vi "Autonomous Motor Input.vi"(0 "RotationTarget":dbl, 1 "Y_axis":dbl, 2 "X_axis":dbl, 5 "Squeeze":dbl, 7 "Cluster in":T1, 9 "Arms":dbl, 12 "ArmLift":dbl, 13 "Hands":dbl, 14 "Lift":dbl) -> (4 "Cluster out":T1)   [LabVIEW 2017]
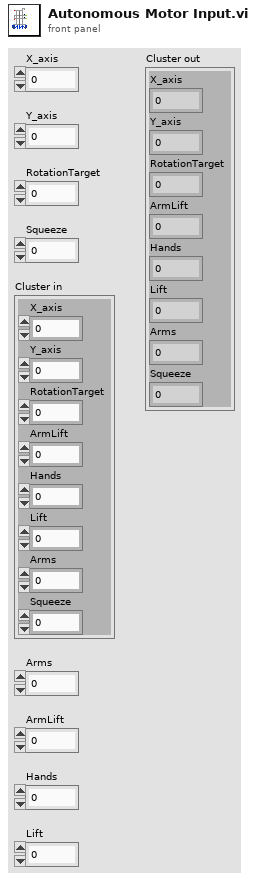
[diagram p1: front panel]
types:
  T1 = cluster{"X_axis":dbl, "Y_axis":dbl, "RotationTarget":dbl, "ArmLift":dbl, "Hands":dbl, "Lift":dbl, "Arms":dbl, "Squeeze":dbl}
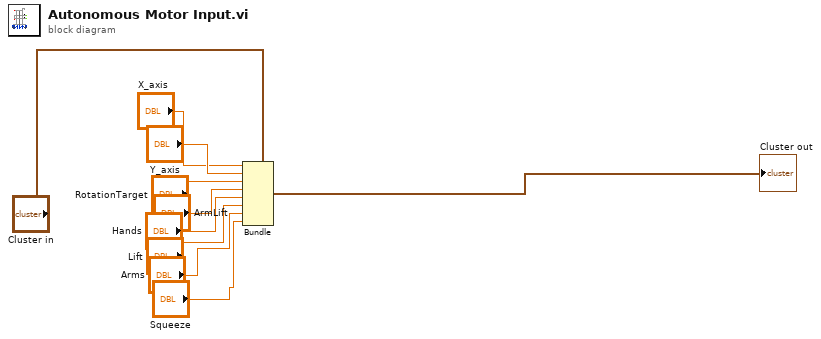
[diagram p0: block diagram]
diagram:
  n1 = Bundle(cluster="Cluster in", "X_axis"="X_axis", "Y_axis"="Y_axis", "RotationTarget"="RotationTarget", "ArmLift"="ArmLift", "Hands"="Hands", "Lift"="Lift", "Arms"="Arms", "Squeeze"="Squeeze") -> (→"Cluster out":T1)
